vi "Obtain Tx to Aircraft Queue Ref.vi"(8 "Error In":errorcluster) -> (0 "error out":errorcluster, 3 "queue out":refnum<queue>)   [LabVIEW 2014]
uses:
  Ground Station to Aircraft Coms/SubVI/Aircraft Data Router/SubVI/Queue References/SubVI/Get Aircraft TX Queue String.vi
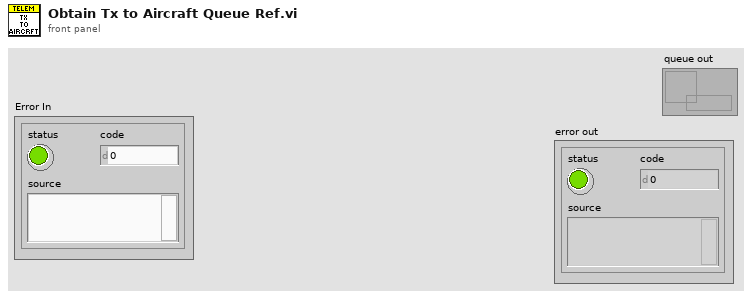
[diagram p1: front panel]
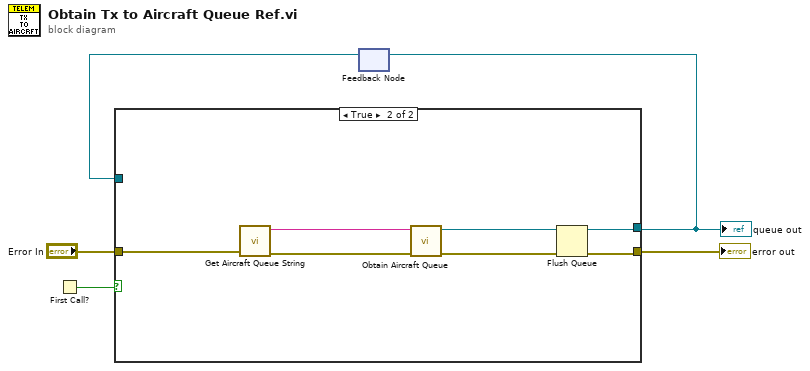
[diagram p0: block diagram]
diagram:
  n1 = First Call?() -> (First Call?: T/F=w4:bool)
  n2 = feedback #1() -> (w2:refnum<queue>)  [unwired: 1 in]
  n3 = case shown="True" w4 {
    tunnel: "Error In" -> [w6 w8]
    tunnel: [w7 w10] -> w3
    tunnel: [w6 w9] -> w1
    tunnel: w2 -> [w7 _]
    frame False {
    }
    frame True {
      n4 = call-poly "Get Aircraft Queue String.vi"("Error In"=w8) -> ("Error Out"=w11:errorcluster, "Aircraft Queue Name"=w14:string)  [unwired: 9 in]
      n5 = call "Obtain Aircraft Queue.vi"("error in (no error)"=w11, "Queue Name"=w14) -> ("error out"=w13:errorcluster, "queue out"=w12:refnum<queue>)  [unwired: 8 in]
      n6 = Flush Queue(queue=w12, error in (no error)=w13) -> (queue out=w10:refnum<queue>, error out=w9:errorcluster)  [unwired: 1 out]
    }
  }
  "error out" <- w1
  "queue out" <- w3
  n7 = feedback-in #1(w3) -> ()
